vi "Advanced Cut - Filter Snippet.vi"(8 "error in (no error)":errorcluster, 10 "Include?":bool, 11 "Snippet in":dbl[](array[numeric])) -> (0 "error out":errorcluster, 2 "Pass?":bool, 3 "Snippet out":dbl[](array[numeric]))   [LabVIEW 2016]
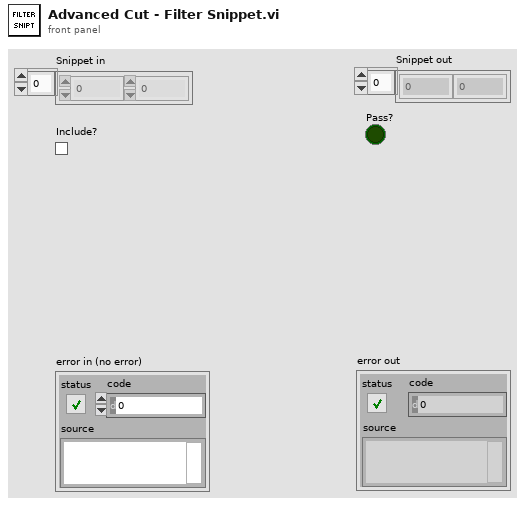
[diagram p1: front panel]
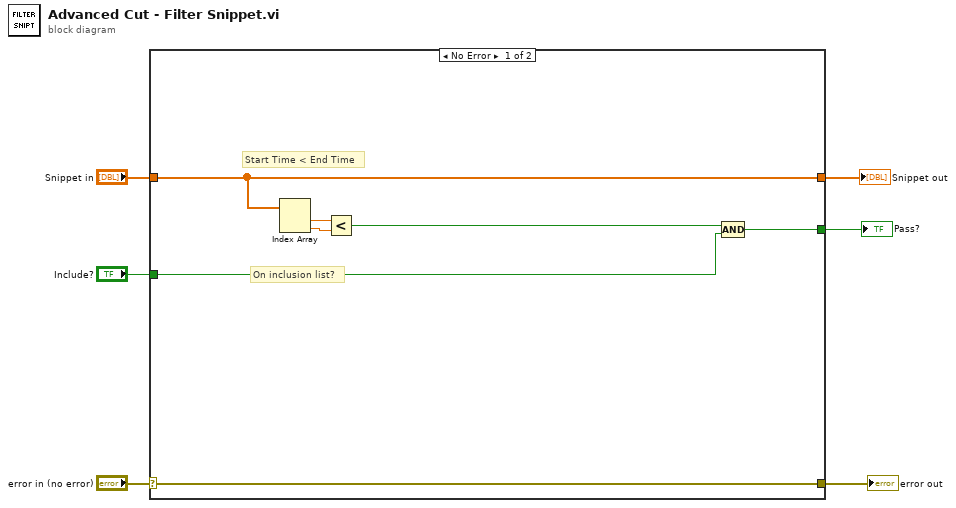
[diagram p0: block diagram]
diagram:
  n1 = case shown="No Error" "error in (no error)" {
    selector: "error in (no error)" -> [w11 w14]
    tunnel: "Snippet in" -> [w13 w15]
    tunnel: [w13 w15] -> w4
    tunnel: "Include?" -> [w12 _]
    tunnel: [w11 w14] -> w3
    tunnel: [w7 _] -> w1
    frame No Error {
      # "On inclusion list?"
      # "Start Time < End Time"
      n2 = Index Array(array=w13) -> (element #1=w9:dbl, element #2=w10:dbl)  [unwired: 2 in]
      n3 = Less?(x=w9, y=w10) -> (x < y?=w8:bool)
      n4 = Compound Arithmetic op=AND(w8, w12) -> (w7:bool)
    }
    frame Error {
    }
  }
  "Snippet out" <- w4
  "error out" <- w3
  "Pass?" <- w1
